vi "Periodic Tasks2.vi"(8 "error in":errorcluster) -> ()   [LabVIEW 2018]
doc: "This VI runs in parallel to other tasks. It can contain as many user-defined periodic loops as you need. These can carry out PID or other sorts of timed response."
uses:
  <vilib>/Rock Robotics/WPI/Utilities/WPI_GetSetVariantRefNum.vi
  Robot Global Data.vi
  <vilib>/Rock Robotics/Network Tables/NT Write Numeric Array.vi
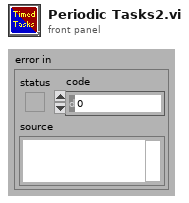
[diagram p1: front panel]
types:
  T1 = typedef "WPI_JoystickDevRef.ctl" = cluster{"Device":T2}
  T2 = typedef "WPI_JoystickDeviceEnum.ctl" = enum16{"USB 0", "USB 1", "USB 2", "USB 3", "USB 4", "USB 5"}
  T3 = typedef "WPI_RobotDriveDevRef.ctl" = cluster{"DevStatus":errorcluster, "Motors[]":T4[], "Square Inputs":bool, "Max Output":dbl}
  T4 = typedef "WPI_MotorControlDeviceRef.ctl" = cluster{"DeviceStatus":errorcluster, "Type":T5, "PWM":cluster{"PWM Channel":T6, "DeadBand":T7}, "CAN":cluster{"Device Number":u8, "SetOutput VI Ref":variant, "GetOutput VI Ref":variant, "Enable VI Ref":variant, "Disable VI Ref":variant, "Data":variant}, "Invert":bool, "DIO PWM":cluster{"PWM \"Enable\" Channel":T6, "DIOChannel":T8, "PWM Rate":dbl}}
  T5 = typedef "WPI_MotorControlType.ctl" = enum16{"PWM", "CAN", "DIO PWM"}
  T6 = typedef "FPGA_DIOPWMChannel.ctl" = enum8{"PWM 0", "PWM 1", "PWM 2", "PWM 3", "PWM 4", "PWM 5", "PWM 6", "PWM 7", "PWM 8", "PWM 9", "PWM MXP 0", "PWM MXP 1", "PWM MXP 2", "PWM MXP 3", "PWM MXP 4", "PWM MXP 5", "PWM MXP 6", "PWM MXP 7", "PWM MXP 8", "PWM MXP 9", "Invalid"}
  T7 = typedef "WPI_PWMDeadband.ctl" = cluster{"Name":string, "maxPositivePwm":i32, "minPositivePwm":i32, "centerPwm":i32, "maxNegativePwm":i32, "minNegativePwm":i32, "angularRange":u16}
  T8 = typedef "FPGA_DIOChannel.ctl" = enum8{"DIO 0", "DIO 1", "DIO 2", "DIO 3", "DIO 4", "DIO 5", "DIO 6", "DIO 7", "DIO 8", "DIO 9", "DIO MXP 0", "DIO MXP 1", "DIO MXP 2", "DIO MXP 3", "DIO MXP 4", "DIO MXP 5", "DIO MXP 6", "DIO MXP 7", "DIO MXP 8", "DIO MXP 9", "DIO MXP 10", "DIO MXP 11", "DIO MXP 12", "DIO MXP 13", "DIO MXP 14", "DIO MXP 15", "SPI Port CS1", "SPI Port CS2", "SPI Port CS3", "SPI Port MISO", "SPI Port MOSI", "Invalid"}
  T9 = cluster{"JoystickDevRef":T1, "RobotDriveDevRef":T3}
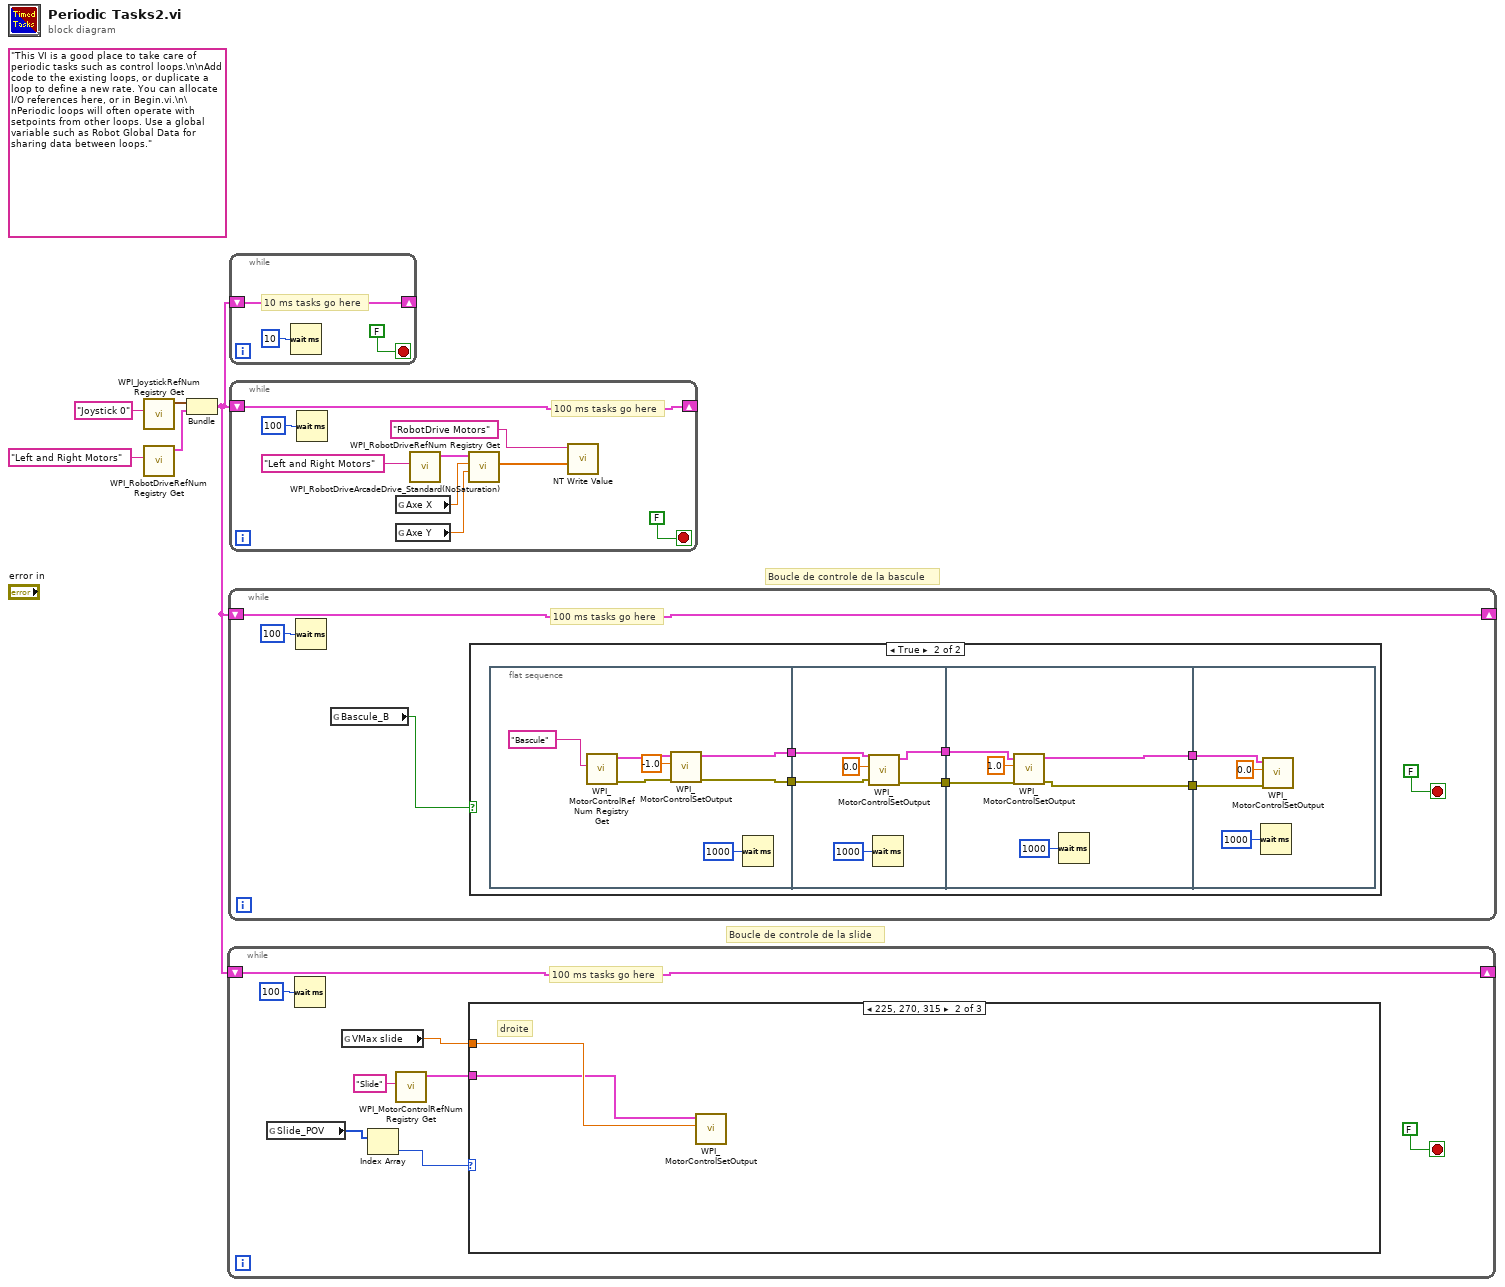
[diagram p0: block diagram]
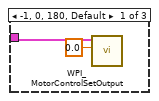
[diagram p2: hidden frame]
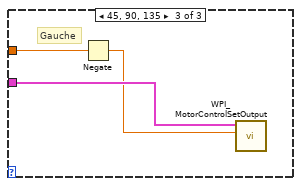
[diagram p3: hidden frame]
diagram:
  (unwired) "This VI is a good place to take care of periodic tasks such as control loops.\n\nAdd code to the existing loops, or duplicate a loop to define a new rate. You can allocate I/O references here, or in Begin.vi.\n\nPeriodic loops will often operate with setpoints from other loops. Use a global variable such as Robot Global Data for sharing data between loops."
  # "Boucle de controle de la slide"
  # "Boucle de controle de la bascule"
  n1 = call <vilib>:"WPI_JoystickRefNum Registry Get.vi"("refnum name"="Joystick 0") -> ("JoystickDevRef"=w3:T1)  [unwired: 1 in, 9 out]
  n2 = call <vilib>:"WPI_RobotDriveRefNum Registry Get.vi"("refnum name"="Left and Right Motors") -> ("RobotDriveDevRef"=w2:T3)  [unwired: 1 in, 9 out]
  n3 = Bundle("JoystickDevRef"=w3, "RobotDriveDevRef"=w2) -> (w1:T9)  [unwired: 1 out]
  n4 = while {
    shift-right: [w11] -> _
    shift-left: w1 -> [w11]
    stop <- FALSE stop-if-true
    # "100 ms tasks go here"
    n5 = global read "Robot Global Data.vi" "Slide_POV"() -> (w10:i16[])
    n6 = Wait (ms)(milliseconds to wait=u32 100) -> ()  [unwired: 1 out]
    n7 = global read "Robot Global Data.vi" "VMax slide"() -> (w6:dbl)
    n8 = Index Array(array=w10) -> (element=w9:i16)  [unwired: 1 in]
    n9 = call <vilib>:"WPI_MotorControlRefNum Registry Get.vi"("refnum name"="Slide") -> ("MotorControlDevRef"=w7:T4)  [unwired: 9 in, 1 out]
    n10 = case shown="225, 270, 315" w9 {
      tunnel: w7 -> [w15 w16 w19]
      tunnel: w6 -> [_ w17 w20]
      frame -1, 0, 180, Default {
        n11 = call <vilib>:"WPI_MotorControlSetOutput.vi"("Output"=0.0, "MotorControlDevRef"=w15) -> ()  [unwired: 7 in, 3 out]
      }
      frame 225, 270, 315 {
        # "droite"
        n12 = call <vilib>:"WPI_MotorControlSetOutput.vi"("Output"=w17, "MotorControlDevRef"=w16) -> ()  [unwired: 7 in, 3 out]
      }
      frame 45, 90, 135 {
        # "Gauche"
        n13 = Negate(x=w20) -> (-x=w18:dbl)
        n14 = call <vilib>:"WPI_MotorControlSetOutput.vi"("Output"=w18, "MotorControlDevRef"=w19) -> ()  [unwired: 7 in, 3 out]
      }
    }
  }
  n15 = while {
    shift-right: [w22] -> _
    shift-left: w1 -> [w22]
    stop <- FALSE stop-if-true
    # "100 ms tasks go here"
    n16 = Wait (ms)(milliseconds to wait=u32 100) -> ()  [unwired: 1 out]
    n17 = global read "Robot Global Data.vi" "Bascule_B"() -> (w21:bool)
    n18 = case shown="True" w21 {
      frame False {
      }
      frame True {
        n19 = flat-sequence {
          tunnel: [w33] -> w30
          tunnel: [w32] -> w27
          tunnel: w30 -> [w42]
          tunnel: [w41] -> w29
          tunnel: w27 -> [w40]
          tunnel: [w39] -> w26
          tunnel: w29 -> [w48]
          tunnel: [w47] -> w28
          tunnel: w26 -> [w46]
          tunnel: [w45] -> w25
          tunnel: w28 -> [w52]
          tunnel: w25 -> [w51]
          frame #0 {
            n20 = call <vilib>:"WPI_MotorControlRefNum Registry Get.vi"("refnum name"="Bascule") -> ("error out"=w36:errorcluster, "MotorControlDevRef"=w37:T4)  [unwired: 9 in]
            n21 = call <vilib>:"WPI_MotorControlSetOutput.vi"("error in (no error)"=w36, "Output"=-1.0, "MotorControlDevRef"=w37) -> ("error out"=w32:errorcluster, "MotorControlDevRef"=w33:T4)  [unwired: 6 in, 1 out]
            n22 = Wait (ms)(milliseconds to wait=u32 1000) -> ()  [unwired: 1 out]
          }
          frame #1 {
            n23 = call <vilib>:"WPI_MotorControlSetOutput.vi"("error in (no error)"=w40, "Output"=0.0, "MotorControlDevRef"=w42) -> ("error out"=w39:errorcluster, "MotorControlDevRef"=w41:T4)  [unwired: 6 in, 1 out]
            n24 = Wait (ms)(milliseconds to wait=u32 1000) -> ()  [unwired: 1 out]
          }
          frame #2 {
            n25 = call <vilib>:"WPI_MotorControlSetOutput.vi"("error in (no error)"=w46, "Output"=1.0, "MotorControlDevRef"=w48) -> ("error out"=w45:errorcluster, "MotorControlDevRef"=w47:T4)  [unwired: 6 in, 1 out]
            n26 = Wait (ms)(milliseconds to wait=u32 1000) -> ()  [unwired: 1 out]
          }
          frame #3 {
            n27 = Wait (ms)(milliseconds to wait=u32 1000) -> ()  [unwired: 1 out]
            n28 = call <vilib>:"WPI_MotorControlSetOutput.vi"("error in (no error)"=w51, "Output"=0.0, "MotorControlDevRef"=w52) -> ()  [unwired: 6 in, 3 out]
          }
        }
      }
    }
  }
  n29 = while {
    shift-right: [w54] -> _
    shift-left: w1 -> [w54]
    stop <- FALSE stop-if-true
    # "10 ms tasks go here"
    n30 = Wait (ms)(milliseconds to wait=u32 10) -> ()  [unwired: 1 out]
  }
  n31 = while {
    shift-right: [w63] -> _
    shift-left: w1 -> [w63]
    stop <- FALSE stop-if-true
    # "100 ms tasks go here"
    n32 = Wait (ms)(milliseconds to wait=u32 100) -> ()  [unwired: 1 out]
    n33 = global read "Robot Global Data.vi" "Axe X"() -> (w57:dbl)
    n34 = global read "Robot Global Data.vi" "Axe Y"() -> (w58:dbl)
    n35 = call <vilib>:"WPI_RobotDriveRefNum Registry Get.vi"("refnum name"="Left and Right Motors") -> ("RobotDriveDevRef"=w61:T3)  [unwired: 1 in, 9 out]
    n36 = call <vilib>:"WPI_RobotDriveArcadeDrive_Standard(NoSaturation).vi"("Y axis value"=w58, "X axis value"=w57, "RobotDriveDevRef"=w61) -> ("Motor Values"=w60:dbl[])  [unwired: 1 in, 7 out]
    n37 = call-poly <vilib>:"NT Write Value.vi"("Numeric Array"=w60, "Name"="RobotDrive Motors") -> ()  [unwired: 9 in, 1 out]
  }
